vi "Create Job VI from Template.vi"() -> ()   [LabVIEW 2013]
uses:
  JobCreatorData -- cluster.ctl
panel:
  in  "Cron Job Templates":i32(listbox)
  in  "Instantiate Job":bool
  # "Select a Cron Job Template for instantiation"
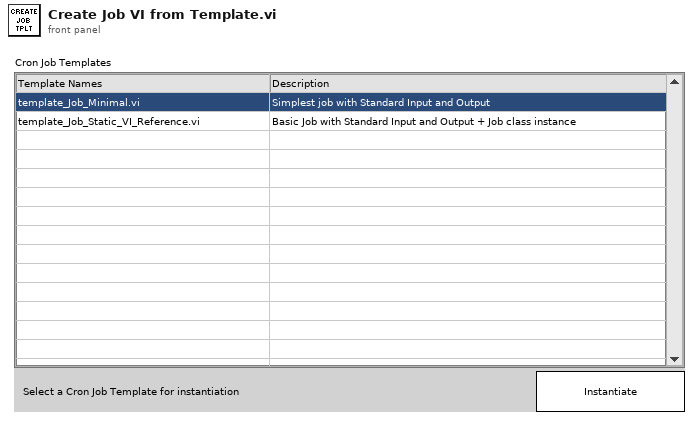
[diagram p1: front panel]
types:
  T1 = enum16{"Initialize", "Discover Template", "Idle", "Create Template", "Exit"}
  T2 = enum32{"Invalid", "Standard", "Closed", "Hidden", "Minimized", "Maximized"}
  T3 = cluster{"App Instance":refnum<vi>, "Active Project":refnum<vi>, "templates":variant, "Cron Folder":path}
  T4 = enum8{"Enabled", "Disabled", "Disabled and Grayed Out"}
  T5 = typedef "JobCreatorData -- cluster.ctl" = cluster{"Path":path, "Name":string, "Description":string}
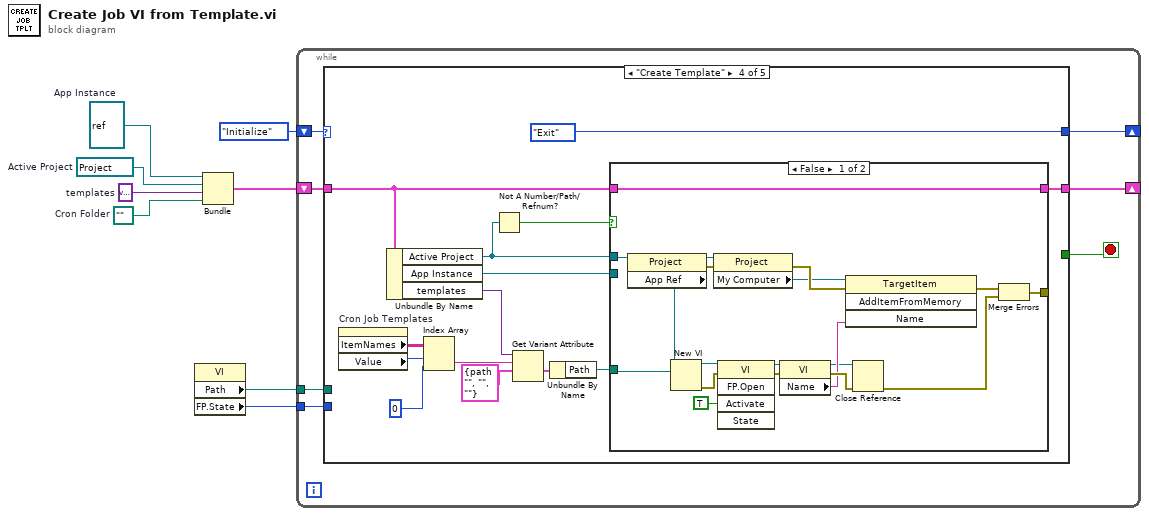
[diagram p0: block diagram]
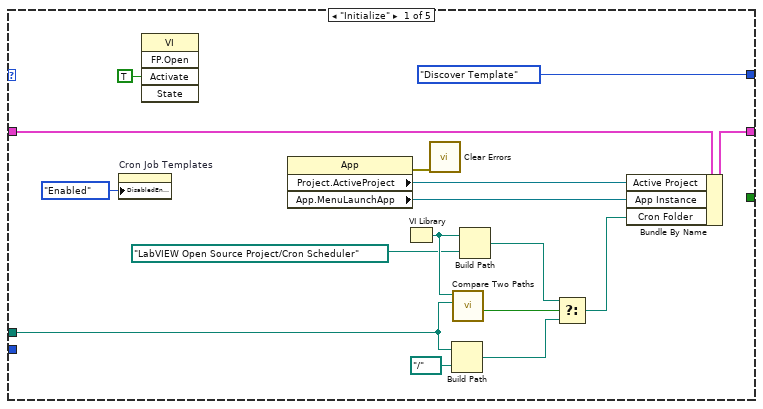
[diagram p2: hidden frame]
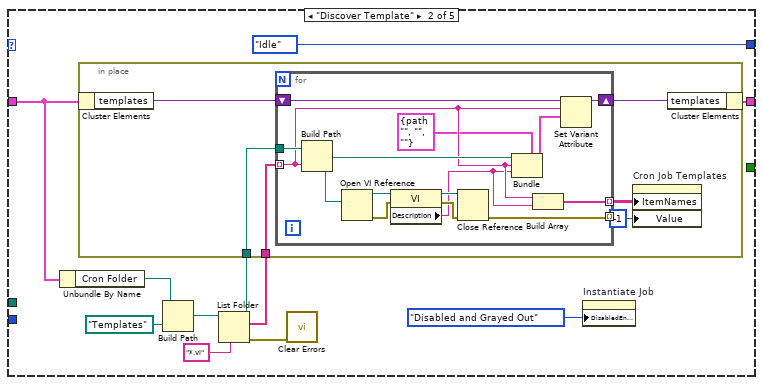
[diagram p3: hidden frame]
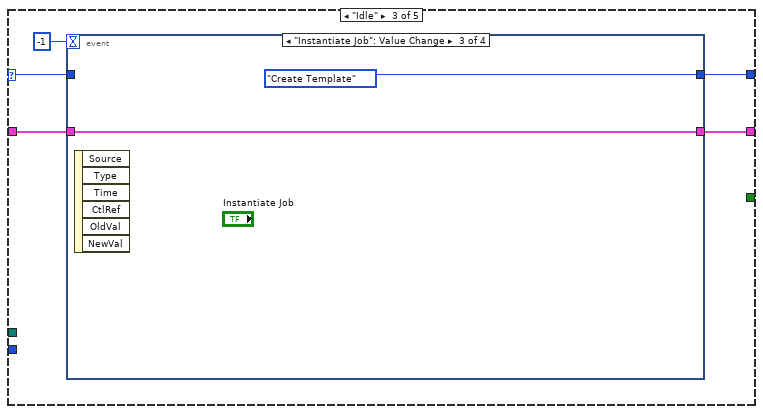
[diagram p4: hidden frame]
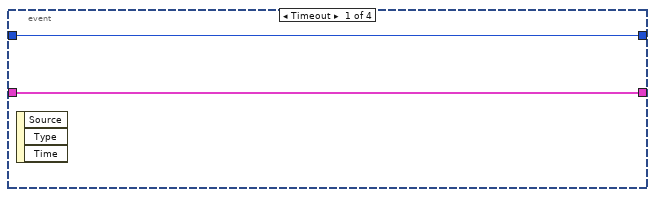
[diagram p5: hidden frame]
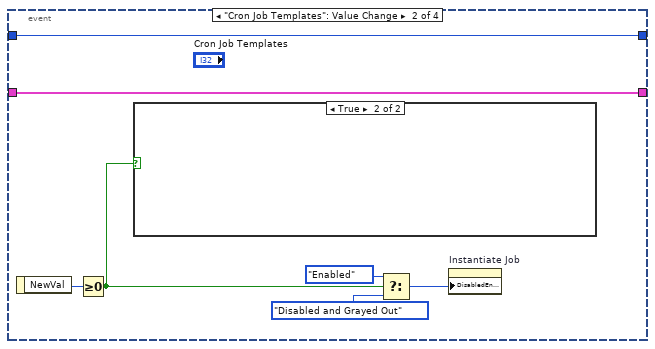
[diagram p6: hidden frame]
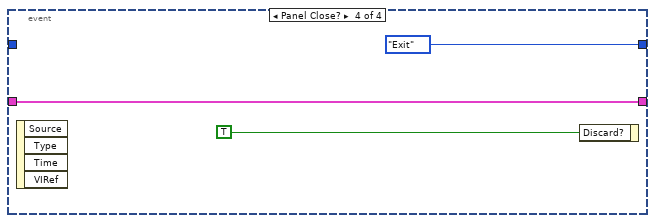
[diagram p8: hidden frame]
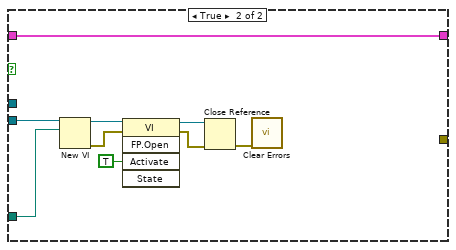
[diagram p9: hidden frame]
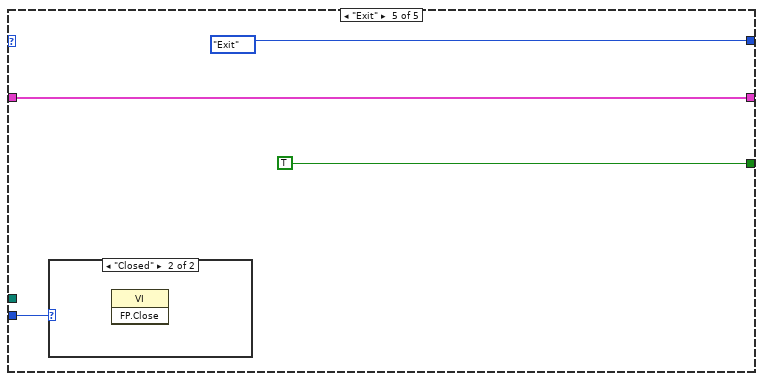
[diagram p10: hidden frame]
diagram:
  w7 = path ""  # Cron Folder
  w6 = variant  # templates
  w5 = refnum<vi> refnum  # App Instance
  w3 = refnum<vi> refnum  # Active Project
  n1 = property class="VI"() -> ("Path"=w1:path, "FP.State"=w2:T2)  [unwired: 2 in, 2 out]
  n2 = Bundle("App Instance"=w5, "Active Project"=w3, "templates"=w6, "Cron Folder"=w7) -> (w4:T3)  [unwired: 1 in]
  n3 = while {
    shift-right: [w14] -> _
    shift-left: T1."Initialize" -> [w15]
    shift-right: [w12] -> _
    shift-left: w4 -> [w13]
    tunnel: w2 -> [w10]
    tunnel: w1 -> [w9]
    stop <- w11 stop-if-true
    n4 = case shown="\"Create Template\"" w15 {
      selector: w15 -> [_ _ w63 _ _]
      tunnel: [T1."Discover Template" T1."Idle" w66 T1."Exit" T1."Exit"] -> w14
      tunnel: w13 -> [w29 w39 w65 w86 w126]
      tunnel: [w30 w41 w64 w85 w126] -> w12
      tunnel: [_ _ _ _ TRUE] -> w11
      tunnel: w10 -> [_ _ _ _ w124]
      tunnel: w9 -> [w25 _ _ _ _]
      frame "Initialize" {
        n5 = property on="Cron Job Templates" class="MCListbox (strict)"("DisabledEnum"=T4."Enabled" ("Disabled")) -> ()  [unwired: 2 in, 2 out]
        n6 = invoke class="VI" method="FP.Open"("Activate"=TRUE ("Activate?")) -> ()  [unwired: 4 in, 5 out]
        n7 = property class="App"() -> (error out=w28:errorcluster, "Project.ActiveProject"=w22:refnum<vi>, "App.MenuLaunchApp"=w27:refnum<vi>)  [unwired: 2 in, 1 out]
        n8 = VI Library() -> (path=w19:path)
        n9 = call <vilib>:"Clear Errors.vi"("error in (no error)"=w28) -> ()  [unwired: 6 in, 1 out]
        n10 = Build Path(base path=w25, name or relative path=path "../.." ("VI Path")) -> (appended path=w23:path)
        n11 = call <vilib>:"Compare Two Paths.vi"("Path 2"=w25, "Path 1"=w19) -> ("Path 2 Relative to Path 1?"=w24:bool)  [unwired: 6 in, 3 out]
        n12 = Build Path(base path=w19, name or relative path=path "LabVIEW Open Source Project/Cron Scheduler" ("VI Path")) -> (appended path=w18:path)
        n13 = Select(t=w18, s=w24, f=w23) -> (s? t:f=w20:path)
        n14 = Bundle By Name(cluster=w29, "Active Project"=w22, "App Instance"=w27, "Cron Folder"=w20) -> (w30:T3)
      }
      frame "Discover Template" {
        n15 = Unbundle By Name(w39) -> ("Cron Folder"=w38:path)
        n16 = Build Path(base path=w38, name or relative path=path "Templates" ("VI Path")) -> (appended path=w37:path)
        n17 = List Folder(path=w37, pattern="*.vi") -> (path out=w34:path, filenames=w35:string[], error out=w33:errorcluster)  [unwired: 2 in, 1 out]
        n18 = in-place {
          in-place-border: w35 -> [w46]
          in-place-border: w34 -> [w45]
          n19 = in-place-cluster #1(w39) -> ("templates"=w48:variant)
          n20 = for {
            tunnel: w46 -> [w52] mode=indexing
            tunnel: w45 -> [w60]
            tunnel: [w55] -> _ mode=indexing
            tunnel: [w50] -> w44 mode=indexing
            shift-right: [w61] -> w47
            shift-left: w48 -> [w62]
            n21 = Build Path(base path=w60, name or relative path=w52) -> (appended path=w58:path)
            n22 = Open VI Reference(vi path=w58) -> (vi reference=w57:refnum<vi>, error out=w54:errorcluster)  [unwired: 5 in]
            n23 = property class="VI"(reference=w57, error in=w54) -> (reference out=w56:refnum<vi>, error out=w53:errorcluster, "Description"=w51:string)
            n24 = Close Reference(reference=w56, error in (no error)=w53) -> (error out=w55:errorcluster)
            n25 = Bundle(cluster=T5 {"Path"=path "", "Name"="", "Description"=""} ("Job Creator Data"), "Path"=w58, "Name"=w52, "Description"=w51) -> (w59:T5)
            n26 = Build Array(w52, w51) -> (w50:string[])
            n27 = Set Variant Attribute(Variant=w62, name=w52, value=w59) -> (Variant out=w61:variant)  [unwired: 1 in, 2 out]
          }
          n28 = property on="Cron Job Templates" class="MCListbox (strict)"("ItemNames"=w44, "Value"=-1 ("Cron Job Templates")) -> ()  [unwired: 2 in, 2 out]
          n29 = in-place-cluster #1("templates"=w47) -> (w41:T3)
        }
        n30 = call <vilib>:"Clear Errors.vi"("error in (no error)"=w33) -> ()  [unwired: 6 in, 1 out]
        n31 = property on="Instantiate Job" class="Bool"("DisabledEnum"=T4."Disabled and Grayed Out" ("Disabled")) -> ()  [unwired: 2 in, 2 out]
      }
      frame "Idle" {
        n32 = event shown="[2] \"Instantiate Job\": Value Change" {
          selector: _ -> [_ _ _ _]
          dyn-events: _ -> [_ _ _ _]
          timeout: -1 -> [_ _ _ _]
          tunnel: [w68 w70 T1."Create Template" T1."Exit"] -> w66
          tunnel: w65 -> [w69 w76 w78 w79]
          tunnel: [w69 w76 w78 w79] -> w64
          tunnel: w63 -> [w68 w70 _ _]
          event Timeout {
            n33 = event-data() -> ()  [unwired: 1 in, 3 out]
          }
          event "Cron Job Templates": Value Change {
            n34 = event-data() -> ("NewVal"=w75:i32)  [unwired: 1 in]
            n35 = Greater Or Equal To 0?(x=w75) -> (x >= 0?=w71:bool)
            n36 = case shown="True" w71 {
              frame False {
              }
              frame True {
              }
            }
            n37 = Select(t=T4."Enabled" ("Disabled"), s=w71, f=T4."Disabled and Grayed Out" ("Disabled")) -> (s? t:f=w72:T4)
            n38 = property on="Instantiate Job" class="Bool"("DisabledEnum"=w72) -> ()  [unwired: 2 in, 2 out]
          }
          event "Instantiate Job": Value Change {
            n39 = event-data() -> ()  [unwired: 1 in, 6 out]
          }
          event Panel Close? {
            n40 = event-data() -> ()  [unwired: 1 in, 4 out]
            n41 = event-data("Discard?"=TRUE) -> ()  [unwired: 1 in, 1 out]
          }
        }
      }
      frame "Create Template" {
        n42 = property on="Cron Job Templates" class="MCListbox (strict)"() -> ("ItemNames"=w94:string[][], "Value"=w92:i32)  [unwired: 2 in, 2 out]
        n43 = Unbundle By Name(w86) -> ("Active Project"=w82:refnum<vi>, "App Instance"=w83:refnum<vi>, "templates"=w90:variant)
        n44 = Index Array(array=w94, index (row)=w92, index (col)=0 ("disabled index (col)")) -> (element=w91:string)
        n45 = Not A Number/Path/Refnum?(number/path/refnum=w82) -> (NaN/Path/Refnum?=w87:bool)
        n46 = Get Variant Attribute(Variant=w90, name=w91, default value (empty Variant)=T5 {"Path"=path "", "Name"="", "Description"=""}) -> (value=w88:T5)  [unwired: 1 in, 3 out]
        n47 = Unbundle By Name(w88) -> ("Path"=w84:path)
        n48 = case shown="False" w87 {
          tunnel: w86 -> [w114 w123]
          tunnel: [w114 w123] -> w85
          tunnel: w84 -> [w96 w116]
          tunnel: w83 -> [_ w117]
          tunnel: w82 -> [w98 _]
          tunnel: [w97 _] -> _
          frame False {
            n49 = property class="Project"(reference=w98) -> (reference out=w102:refnum<vi>, error out=w105:errorcluster, "App Ref"=w101:refnum<vi>)  [unwired: 1 in]
            n50 = New VI(10:w96, 11:w101) -> (0:w108:errorcluster, 3:w100:refnum<vi>)  [unwired: 5 in]
            n51 = property class="Project"(reference=w102, error in=w105) -> (error out=w111:errorcluster, "My Computer"=w103:refnum<vi>)  [unwired: 1 out]
            n52 = invoke class="VI" method="FP.Open"(reference=w100, error in=w108, "Activate"=TRUE ("Activate?")) -> (reference out=w104:refnum<vi>, error out=w109:errorcluster)  [unwired: 2 in, 3 out]
            n53 = property class="VI"(reference=w104, error in=w109) -> (reference out=w106:refnum<vi>, error out=w110:errorcluster, "Name"=w107:string)
            n54 = invoke class="TargetItem" method="AddItemFromMemory"(reference=w103, error in=w111, "Name"=w107) -> (error out=w112:errorcluster)  [unwired: 1 in, 3 out]
            n55 = Close Reference(reference=w106, error in (no error)=w110) -> (error out=w113:errorcluster)
            n56 = Merge Errors(w112, w113) -> (w97:errorcluster)
          }
          frame True {
            n57 = New VI(10:w116, 11:w117) -> (0:w121:errorcluster, 3:w119:refnum<vi>)  [unwired: 5 in]
            n58 = invoke class="VI" method="FP.Open"(reference=w119, error in=w121, "Activate"=TRUE ("Activate?")) -> (reference out=w120:refnum<vi>, error out=w122:errorcluster)  [unwired: 2 in, 3 out]
            n59 = Close Reference(reference=w120, error in (no error)=w122) -> (error out=w115:errorcluster)
            n60 = call <vilib>:"Clear Errors.vi"("error in (no error)"=w115) -> ()  [unwired: 6 in, 1 out]
          }
        }
      }
      frame "Exit" {
        n61 = case shown="\"Closed\"" w124 {
          frame "Invalid", Default {
          }
          frame "Closed" {
            n62 = invoke class="VI" method="FP.Close"() -> ()  [unwired: 3 in, 3 out]
          }
        }
      }
    }
  }
